vi "Configure Power Analysis (Switching Loss).vi"(5 "Voltage Switching Level (5 Percent)":dbl=5.0, 6 "Current Switching Level (5 Percent)":dbl=5.0, 7 "Vcesat (2 V)":dbl=2.0, 8 "error in (no error)":errorcluster, 9 "Rdson (0.02 Ohm)":dbl=0.02, 10 "Conduction Calculation Method (0: Waveform)":i32(ring) items=["Waveform", "Rdson", "Vcesat"], 11 "VISA resource name":refnum<visa-resource-name>) -> (0 "error out":errorcluster, 3 "VISA resource name out":refnum<visa-resource-name>)   [LabVIEW 2015, in "Agilent 2000 3000 X-Series.lvlib"]
doc: "Configures the conduction calculation method, V reference, and I reference settings and applies the switching loss analysis.\n\n<B>Note(s):</B>\nUse <B>Read Measurement (Switching Loss Power Analysis).vi</B> to read the result of this power analysis.\nThis VI is not supported by EDUX1052A/G, DSOX1202A/G, DSOX1204A/G models"
uses:
  Agilent 2000 3000 X-Series.lvlib
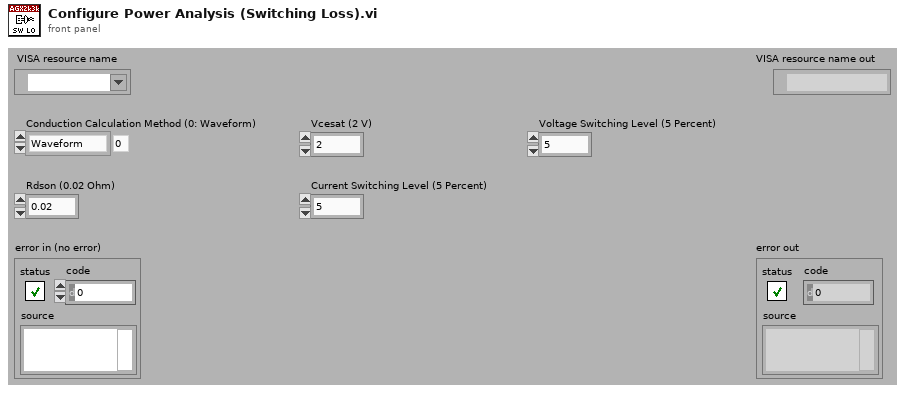
[diagram p1: front panel]
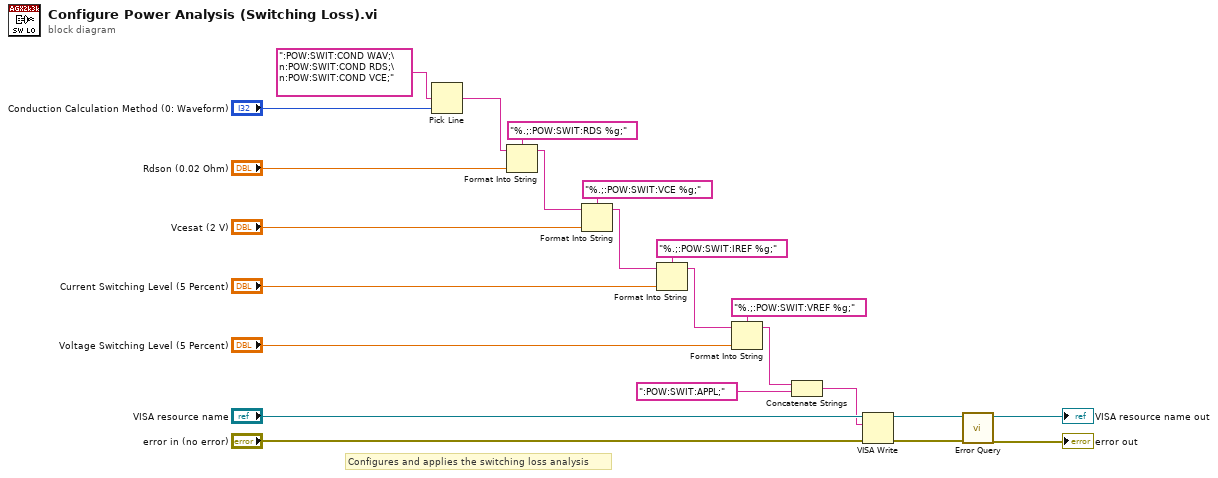
[diagram p0: block diagram]
diagram:
  # "Configures and applies the switching loss analysis"
  n1 = Pick Line(multi-line string=":POW:SWIT:COND WAV;\n:POW:SWIT:COND RDS;\n:POW:SWIT:COND VCE;", line index="Conduction Calculation Method (0: Waveform)") -> (output string=w21:string)  [unwired: 1 out]
  n2 = Format Into String(format string="%.;:POW:SWIT:RDS %g;", initial string=w21, "Rdson (0.02 Ohm)") -> (resulting string=w18:string)  [unwired: 1 in, 1 out]
  n3 = Format Into String(format string="%.;:POW:SWIT:VCE %g;", initial string=w18, "Vcesat (2 V)") -> (resulting string=w15:string)  [unwired: 1 in, 1 out]
  n4 = Format Into String(format string="%.;:POW:SWIT:IREF %g;", initial string=w15, "Current Switching Level (5 Percent)") -> (resulting string=w12:string)  [unwired: 1 in, 1 out]
  n5 = Format Into String(format string="%.;:POW:SWIT:VREF %g;", initial string=w12, "Voltage Switching Level (5 Percent)") -> (resulting string=w2:string)  [unwired: 1 in, 1 out]
  n6 = Concatenate Strings(w2, ":POW:SWIT:APPL;") -> (w1:string)
  n7 = VISA Write(VISA resource name="VISA resource name", write buffer=w1, error in (no error)="error in (no error)") -> (VISA resource name out=w7:refnum<visa-resource-name>, error out=w6:errorcluster)  [unwired: 1 out]
  n8 = call "Error Query.vi"("error in (no error)"=w6, "VISA resource name"=w7) -> ("error out"=→"error out":errorcluster, "VISA resource name out"=→"VISA resource name out":refnum<visa-resource-name>)  [unwired: 8 out]
